vi "Dash_Globals.vi"() -> ()   [LabVIEW 2019]
panel:
  in  "Turret_Zero":dbl
  in  "Flywheel_Table":dbl[][](array[numeric])
  in  "Auto_Selection":string
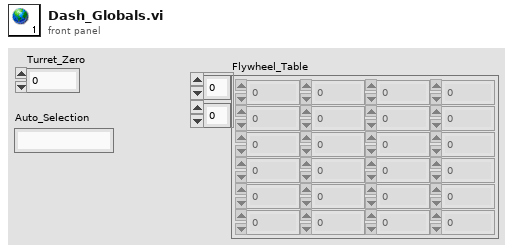
[diagram p1: front panel]
diagram:
